vi "Start Timer.vi"(8 "error in (no error)":errorcluster, 9 "Correlation ID":u32, 10 "Wait Time (s)":dbl, 11 "Application in":refnum<class "Application.lvclass">) -> (0 "error out":errorcluster, 3 "Application out":refnum<class "Application.lvclass">)   [LabVIEW 2023, in "Application.lvlib" / "Application.lvclass"]
uses:
  Application.lvclass
  Application.lvclass/Application.ctl
  Timer Messages/Start Msg/Start Msg.lvclass
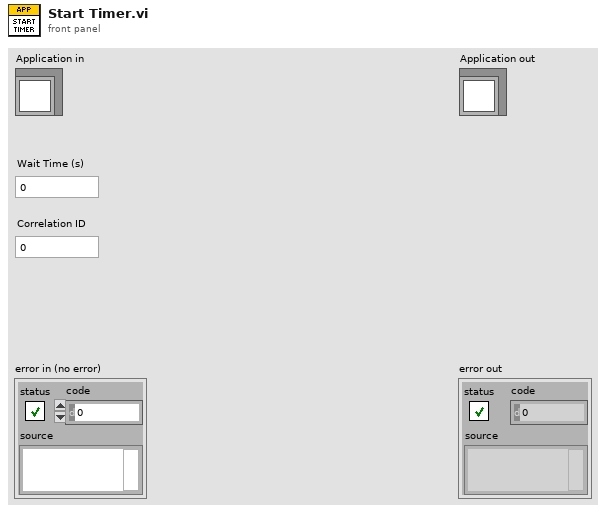
[diagram p1: front panel]
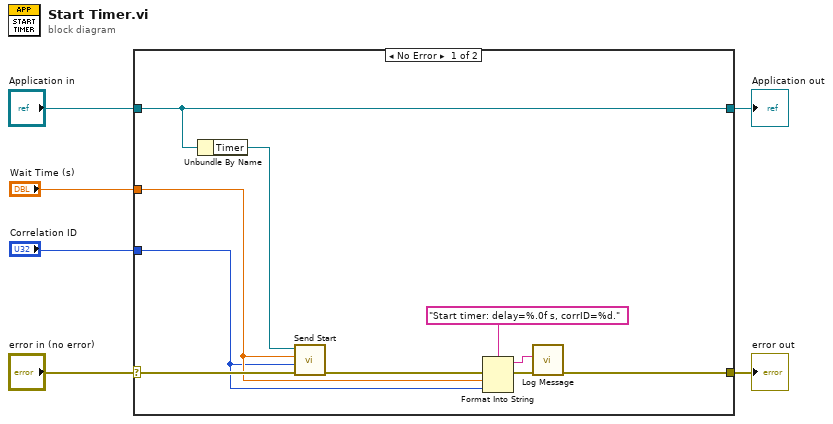
[diagram p0: block diagram]
diagram:
  n1 = case shown="No Error" "error in (no error)" {
    selector: "error in (no error)" -> [w16 w18]
    tunnel: [w11 w18] -> w5
    tunnel: [w8 w17] -> w3
    tunnel: "Application in" -> [w8 w17]
    tunnel: "Wait Time (s)" -> [w10 _]
    tunnel: "Correlation ID" -> [w9 _]
    frame No Error {
      n2 = Unbundle By Name(w8) -> ("Timer"=w7:refnum<class "Message Enqueuer.lvclass">)
      n3 = call "Send Start.vi"("error in (no error)"=w16, "Correlation ID"=w9, "Wait Time (s)"=w10, "Message Enqueuer"=w7) -> ("error out"=w13:errorcluster)  [unwired: 6 in, 1 out]
      n4 = Format Into String(format string="Start timer: delay=%.0f s, corrID=%d.", error in=w13, w10, w9) -> (resulting string=w15:string, error out=w12:errorcluster)  [unwired: 1 in]
      n5 = call "Log Message.vi"("error constant"=w12, "input"=w15) -> ("error constant 2"=w11:errorcluster)  [unwired: 8 in, 1 out]
    }
    frame Error {
    }
  }
  "error out" <- w5
  "Application out" <- w3
